vi "MU Read Chip Revision Of Parameter File.vi"(8 "error in (no error)":errorcluster, 10 "filepath":string, 11 "handle":u64) -> (0 "error out (no error)":errorcluster, 2 "revisionCode":u32, 3 "function return":u32)   [LabVIEW 2017, in "MU_3SL_interface.lvlib"]
uses:
  MU_3SL_interface.lvlib
  lib/MU_3SL_interface.dll
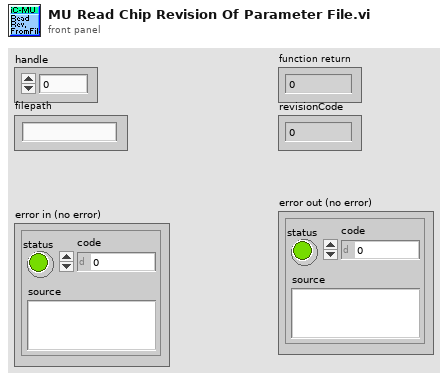
[diagram p1: front panel]
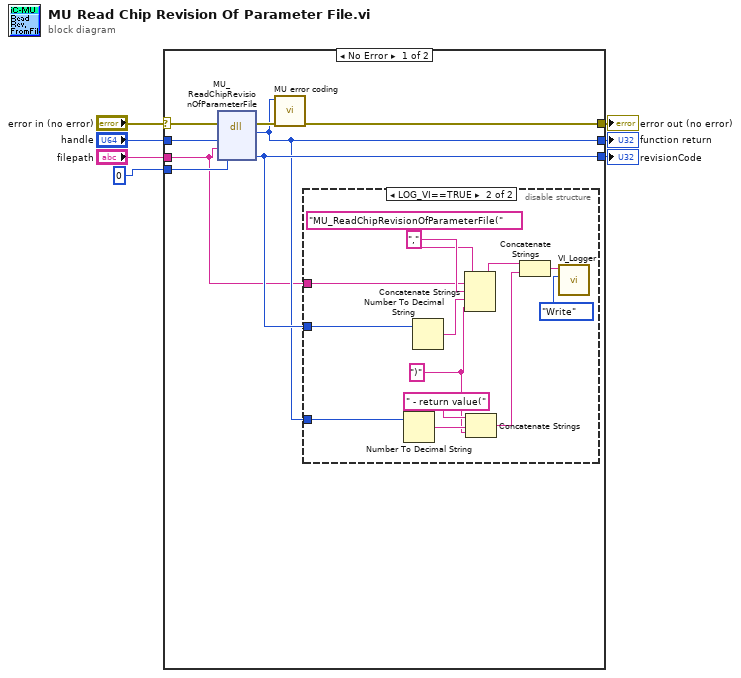
[diagram p0: block diagram]
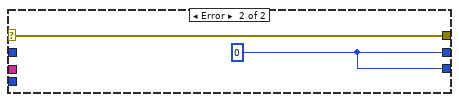
[diagram p3: hidden frame]
diagram:
  n1 = case shown="No Error" "error in (no error)" {
    selector: "error in (no error)" -> [w12 w30]
    tunnel: [w9 w29] -> w7
    tunnel: "handle" -> [w15 _]
    tunnel: "filepath" -> [w8 _]
    tunnel: [w13 w30] -> w4
    tunnel: u32 0 ("revisionCode") -> [w11 _]
    tunnel: [w10 w29] -> w1
    frame No Error {
      n2 = dll-call lib="C:/Users/bes/AppData/Roaming/work/mu_9so/icsubmodules/soft_mu_3sl_master/lv_interface/lib/MU_3SL_interface**.*" fn="MU_ReadChipRevisionOfParameterFile"(error in=w12, "handle"=w15, "filepath"=w8, "revisionCode"=w11) -> (error out=w14:errorcluster, "return type"=w9:u32, "revisionCode"=w10:u32)  [unwired: 4 in, 1 out]
      n3 = call "MU error coding.vi"("error in (no error)"=w14, "function return in"=w9) -> ("error out"=w13:errorcluster)  [unwired: 9 in]
      n4 = disable-structure shown="LOG_VI==TRUE" {
        disable-tunnel: w9 -> [_ w26]
        disable-tunnel: w10 -> [_ w20]
        disable-tunnel: w8 -> [_ w16]
        frame condition #0 {
        }
        frame condition #1 (active) {
          w17 = ")" ("string")
          n5 = Number To Decimal String(number=w26) -> (decimal integer string=w25:string)  [unwired: 1 in]
          n6 = Number To Decimal String(number=w20) -> (decimal integer string=w19:string)  [unwired: 1 in]
          n7 = Concatenate Strings("MU_ReadChipRevisionOfParameterFile(" ("Info in"), w16, "," ("string"), w19, w17) -> (w24:string)
          n8 = Concatenate Strings(" - return value(" ("string"), w25, w17) -> (w23:string)
          n9 = Concatenate Strings(w24, w23) -> (w22:string)
          n10 = call "VI_Logger.vi"("Action (Read)"=enum16{"Write", "Read"}."Write", "Info in"=w22) -> ()  [unwired: 8 in, 2 out]
        }
      }
    }
    frame Error {
      w29 = u32 0
    }
  }
  "function return" <- w7
  "error out (no error)" <- w4
  "revisionCode" <- w1
